vi "Test Save QOI (Memory).vi"(8 "error in (no error)":errorcluster) -> (0 "error out":errorcluster, 3 "Pass?":bool)   [LabVIEW 2020]
uses:
  <vilib>/picture/picture.llb/imagedata.ctl
  G-Image/Image IO/Polymorphic VIs/Save BMP Image (Memory).vi/3f50d8b1-806b-44de-96ec-55f047b16f0f.vi
  G-Image/Private/Result To Error.vi
  G-Image/Private/Get Image Data.vi
  G-Image/Private/ARGB To RGBA.vi
  G-Image/Private/Depth To Number Channels.vi
  G-Image/Image Processing/Indexed Color To True Color Image.vi
  <vilib>/Utility/error.llb/Error Cluster From Error Code.vi
  G-Image/Image IO/Polymorphic VIs/Load Image (Memory).vi
  G-Image/G-Image.lvlib
  G-Image/Image IO/Polymorphic VIs/Save QOI Image (Memory).vi
panel:
  out "Array":cluster{string, "new picture":picture}[](array[cluster])
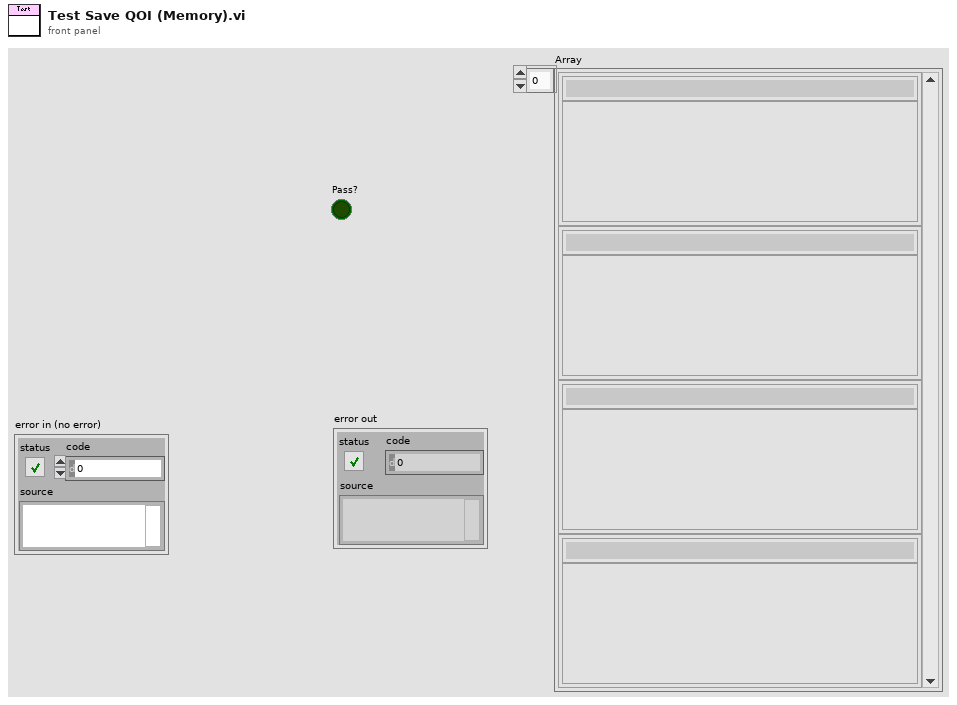
[diagram p1: front panel]
types:
  T1 = typedef "imagedata.ctl" = cluster{"image type":i32, "image depth":i32, "image":u8[], "mask":u8[], "colors":u32[], "Rectangle":cluster{"left":i16, "top":i16, "right":i16, "bottom":i16}}
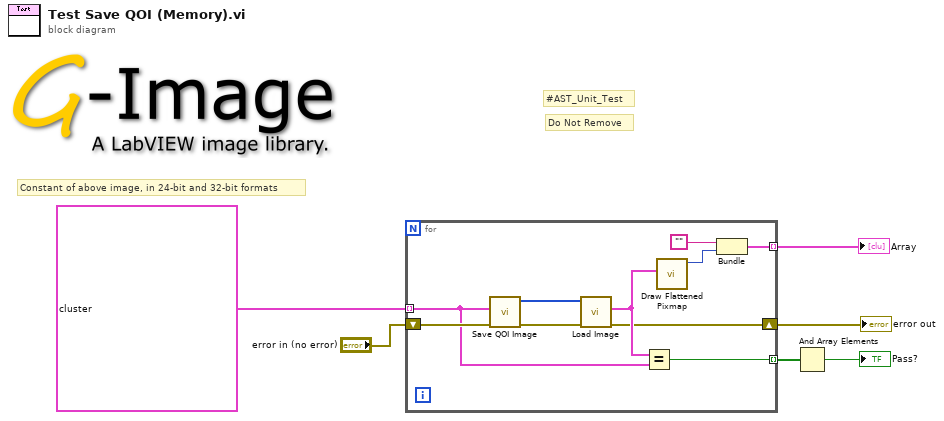
[diagram p0: block diagram]
diagram:
  # "Constant of above image, in 24-bit and 32-bit formats"
  # "Do Not Remove"
  # "#AST_Unit_Test"
  n1 = for {
    tunnel: T1[] [{"image type"=0, "image depth"=24, "image"=array[115500 elements], "mask"=[], "colors"=[], "Rectangle"={"left"=0, "top"=0, "right"=350, "bottom"=110}}, {"image type"=0, "image depth"=32, "image"=array[154000 elements], "mask"=array[4840 elements], "colors"=[], "Rectangle"={"left"=0, "top"=0, "right"=350, "bottom"=110}}] ("Array 2") -> [w13] mode=indexing
    shift-right: [w8] -> w4
    shift-left: "error in (no error)" -> [w16]
    tunnel: [w12] -> w3 mode=indexing
    tunnel: [w9] -> w5 mode=indexing
    n2 = call-poly "Save QOI Image.vi"("error in (no error)"=w16, "Image"=w13) -> ("error out"=w14:errorcluster, "Encoded Image"=w15:u8[])  [unwired: 8 in]
    n3 = call-poly "Load Image.vi"("error in (no error)"=w14, "Encoded Image"=w15) -> ("error out"=w8:errorcluster, "Image"=w11:T1)  [unwired: 8 in]
    n4 = Equal?(x=w11, y=w13) -> (x = y?=w12:bool)
    n5 = call <vilib>:"Draw Flattened Pixmap.vi"("image data"=w11) -> ("new picture"=w10:picture)  [unwired: 8 in]
    n6 = Bundle("", "new picture"=w10) -> (w9:cluster{string, "new picture":picture})  [unwired: 1 in]
  }
  "error out" <- w4
  "Array" <- w5
  n7 = And Array Elements(Boolean array=w3) -> (logical AND=→"Pass?":bool)
